vi "TagVar Data(SGL).vi"(8 "错误输入":errorcluster, 9 "method":T2=enum."读取", 10 "TagData":T1, 11 "TagList":T1[](array[typedef])) -> (0 "错误输出":errorcluster, 1 "TagDataArray":T1[](array[typedef]), 3 "TagData":T1)   [LabVIEW 2013, in "Tag Data by Variant.lvlib"]
uses:
  Tag Data by Variant.lvlib
  Custom def/Tag SGL.ctl
  Custom def/mode.ctl
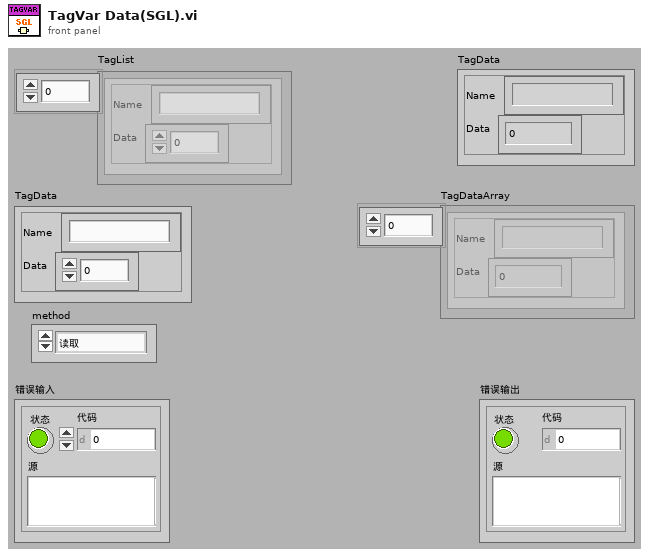
[diagram p1: front panel]
types:
  T1 = typedef "Tag Data by Variant.lvlib/Tag SGL.ctl" = cluster{"Name":string, "Data":sgl}
  T2 = typedef "Tag Data by Variant.lvlib/mode.ctl" = enum16{"初始化", "加入", "删除", "读取", "读取所有", "清除"}
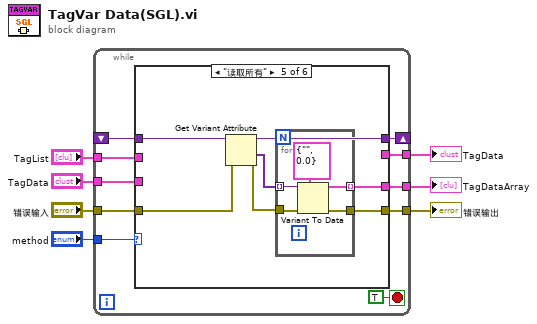
[diagram p0: block diagram]
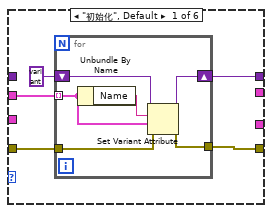
[diagram p2: hidden frame]
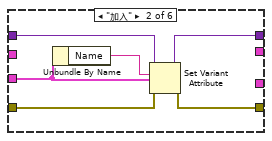
[diagram p3: hidden frame]
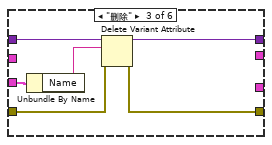
[diagram p4: hidden frame]
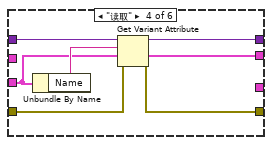
[diagram p5: hidden frame]
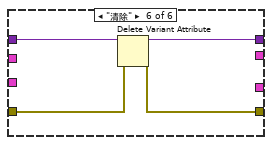
[diagram p6: hidden frame]
diagram:
  n1 = while {
    shift-right: [w14] -> _
    shift-left: _ -> [w10]
    tunnel: "method" -> [w16]
    tunnel: "TagList" -> [w15]
    tunnel: "错误输入" -> [w13]
    tunnel: [w12] -> w4
    tunnel: "TagData" -> [w11]
    tunnel: [w9] -> w2
    tunnel: [w8] -> w1
    stop <- TRUE stop-if-true
    n2 = case shown="\"读取所有\"" w16 {
      tunnel: w15 -> [w21 _ _ _ _ _]
      tunnel: [w18 w31 w39 w46 w53 w62] -> w14
      tunnel: w13 -> [w20 w33 w36 w44 w52 w61]
      tunnel: [w19 w32 w35 w43 w48 w60] -> w12
      tunnel: w11 -> [_ w29 w38 w42 _ _]
      tunnel: w10 -> [_ w34 w40 w47 w54 w63]
      tunnel: [_ _ _ w41 _ _] -> w9
      tunnel: [_ _ _ _ w50 _] -> w8
      frame "初始化", Default {
        n3 = for {
          tunnel: w21 -> [w26] mode=indexing
          tunnel: w20 -> [w25]
          tunnel: [w24] -> w19
          shift-right: [w23] -> w18
          shift-left: variant ("变体") -> [w28]
          n4 = Unbundle By Name(w26) -> ("Name"=w27:string)
          n5 = Set Variant Attribute(Variant=w28, name=w27, value=w26, error in=w25) -> (Variant out=w23:variant, error out=w24:errorcluster)  [unwired: 1 out]
        }
      }
      frame "加入" {
        n6 = Unbundle By Name(w29) -> ("Name"=w30:string)
        n7 = Set Variant Attribute(Variant=w34, name=w30, value=w29, error in=w33) -> (Variant out=w31:variant, error out=w32:errorcluster)  [unwired: 1 out]
      }
      frame "删除" {
        n8 = Unbundle By Name(w38) -> ("Name"=w37:string)
        n9 = Delete Variant Attribute(4:w36, 6:w37, 7:w40) -> (0:w35:errorcluster, 3:w39:variant)  [unwired: 1 out]
      }
      frame "读取" {
        n10 = Unbundle By Name(w42) -> ("Name"=w45:string)
        n11 = Get Variant Attribute(Variant=w47, name=w45, default value (empty Variant)=w42, error in=w44) -> (duplicate Variant=w46:variant, value=w41:T1, error out=w43:errorcluster)  [unwired: 1 out]
      }
      frame "读取所有" {
        n12 = Get Variant Attribute(Variant=w54, error in=w52) -> (duplicate Variant=w53:variant, values=w51:variant[], error out=w49:errorcluster)  [unwired: 2 in, 1 out]
        n13 = for {
          tunnel: w51 -> [w59] mode=indexing
          tunnel: [w58] -> w50 mode=indexing
          tunnel: w49 -> [w57]
          tunnel: [w56] -> w48
          n14 = Variant To Data(error in=w57, type=T1 {"Name"="", "Data"=0.0} ("TagData"), Variant=w59) -> (data=w58:T1, error out=w56:errorcluster)
        }
      }
      frame "清除" {
        n15 = Delete Variant Attribute(4:w61, 7:w63) -> (0:w60:errorcluster, 3:w62:variant)  [unwired: 1 in, 1 out]
      }
    }
  }
  "错误输出" <- w4
  "TagData" <- w2
  "TagDataArray" <- w1
